vi "List Project.vi"(8 "error in (no error)":errorcluster, 11 "Rename in":refnum<class "ProjectItem.lvclass">) -> (0 "error out":errorcluster, 3 "Rename out":refnum<class "ProjectItem.lvclass">)   [LabVIEW 2019, in "ProjectItem.lvclass"]
uses:
  ProjectItem.lvclass
  ProjectItem.lvclass/ProjectItem.ctl
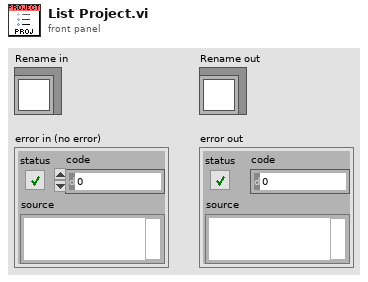
[diagram p1: front panel]
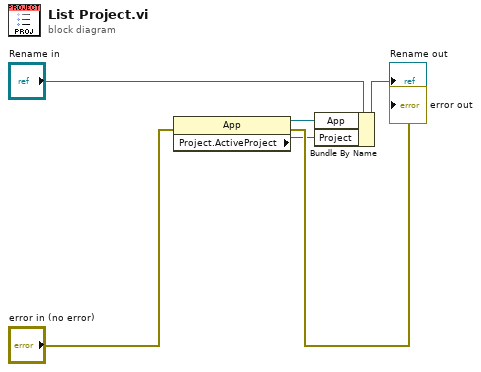
[diagram p0: block diagram]
diagram:
  n1 = property class="App"(error in="error in (no error)") -> (reference out=w2:refnum<vi>, error out=→"error out":errorcluster, "Project.ActiveProject"=w3:refnum<vi>)  [unwired: 1 in]
  n2 = Bundle By Name(cluster="Rename in", "App"=w2, "Project"=w3) -> (→"Rename out":refnum<class "ProjectItem.lvclass">)
